vi "student_receiver.vi"() -> ()   [LabVIEW 2021]
uses:
  <vilib>/sound2/lvsound2.llb/Sound Data Format.ctl
  <vilib>/addons/Modulation/Analog/support/mod_Set Error Source.vi
  <vilib>/addons/Modulation/Digital/Support/Common/Validators/mod_Generate Filter Coefficients Validate.vi
  <vilib>/addons/Modulation/Digital/General/subVIs/mod_Generate Filter Coefficients.vi
  <vilib>/addons/Modulation/Digital/General/MT Generate PSK System Parameters(M).vi
  <instrlib>/niUSRP/niUSRP Fetch Rx Data (CDB Cluster).vi
  <vilib>/sound2/lvsound2.llb/Sound File Info (path).vi
  <vilib>/addons/Modulation/niDMT.lvlib
panel:
  in  "stop 2":bool
  out "data":waveform(dbl)[](array[waveform])
  in  "samples per symbol (16)":i32=16
  in  "differential PSK":enum16{"disable", "enable"}(ring)
  out "sound format":T1={"sample rate (S/s)"=22050.0, "number of channels"=2, "bits per sample"=16}
  in  "matched samples per symbol (16)":i32=16
  in  "Path input":path
  out "Constellation Graph":T2(graph)
  in  "pulse shaping samples per symbol (16)":i32=16
  in  "pulse shaping filter (none)":T3(ring)
  out "coerced gain":dbl format="%#_6f"
  out "coerced carrier frequency":dbl=100000.0 format="%#_6p"
  out "coerced IQ rate":dbl=100000.0 format="%#_6p"
  in  "Recv carrier frequency":dbl=100000.0 format="%#_6p"
  in  "Recv IQ rate":dbl=100000.0 format="%#_6p"
  in  "number of samples":i64=100000
  in  "active antenna 2":string
  in  "gain":dbl format="%#_6f"
  out "error out":errorcluster
  in  "error in (no error)":errorcluster
  in  "USRP IP Address":refnum<k15>
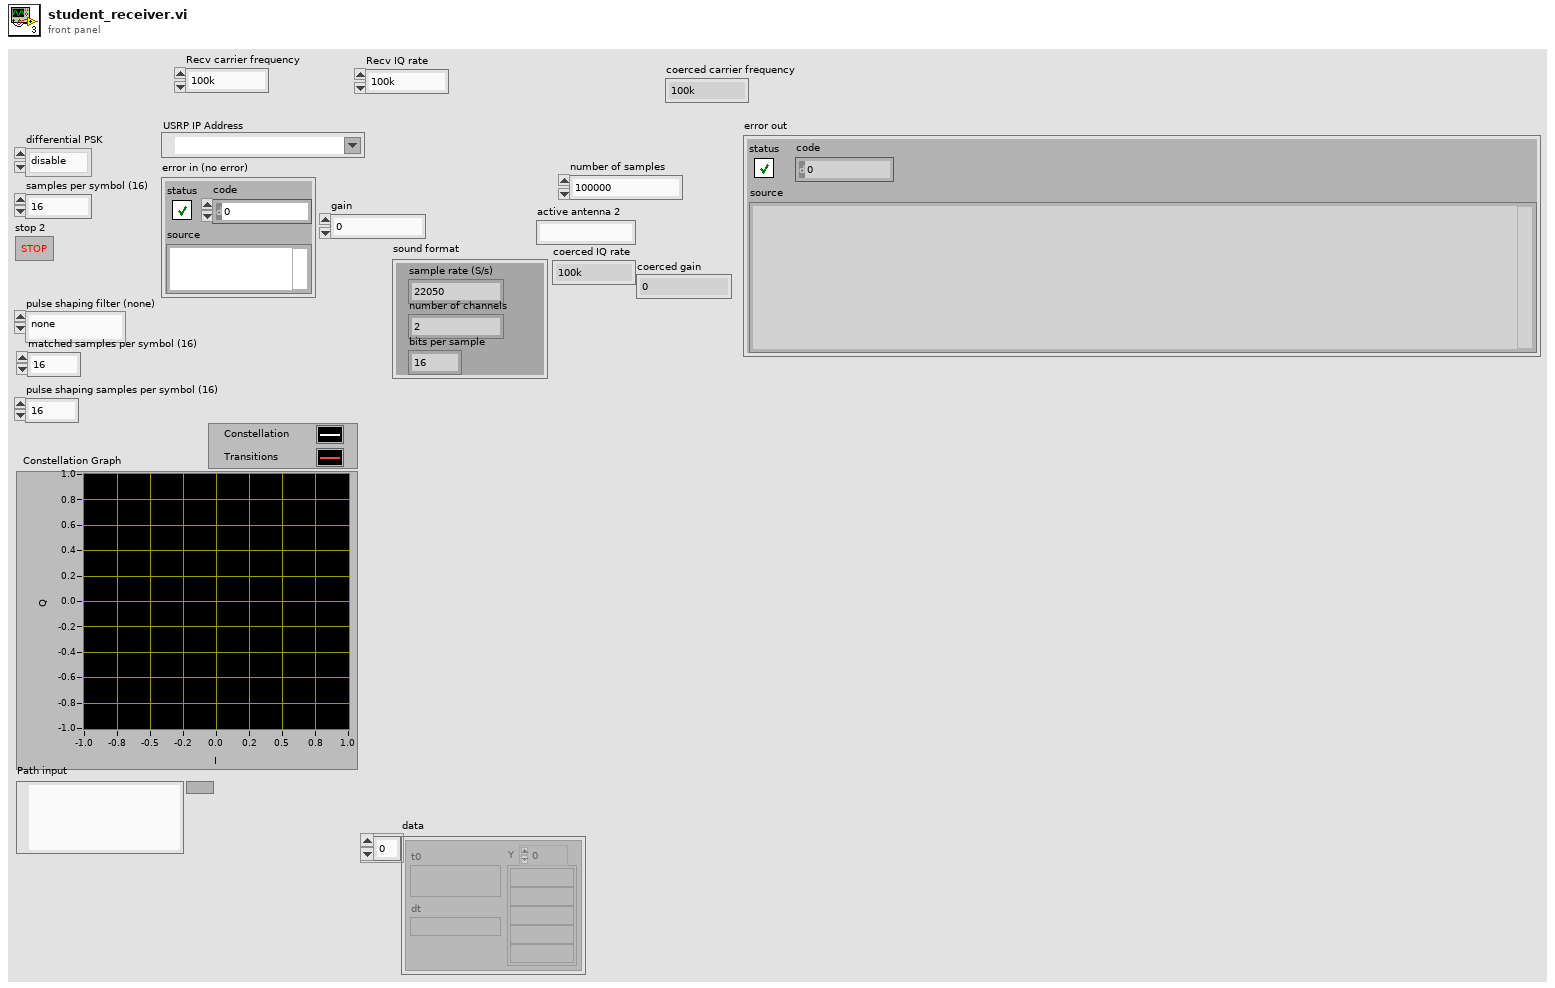
[diagram p1: front panel]
types:
  T1 = typedef "Sound Data Format.ctl" = cluster{"sample rate (S/s)":dbl, "number of channels":i32, "bits per sample":i32}
  T2 = cluster{"Decimated Array":dbl[], "Decimated Array":dbl[]}[]
  T3 = enum16{"none", "Raised Cosine", "Root Raised Cos", "Gaussian"}
  T4 = enum16{"FSK", "PSK", "QAM", "MSK", "PAM", "ASK", "CPM"}
  T5 = cluster{"samples per symbol (16)":i32, "symbol map":cdb[], "differential PSK":enum16{"disable", "enable"}, "PSK type":u16}
  T6 = cluster{"constellation":dbl[], "oversampled data":dbl[]}[]
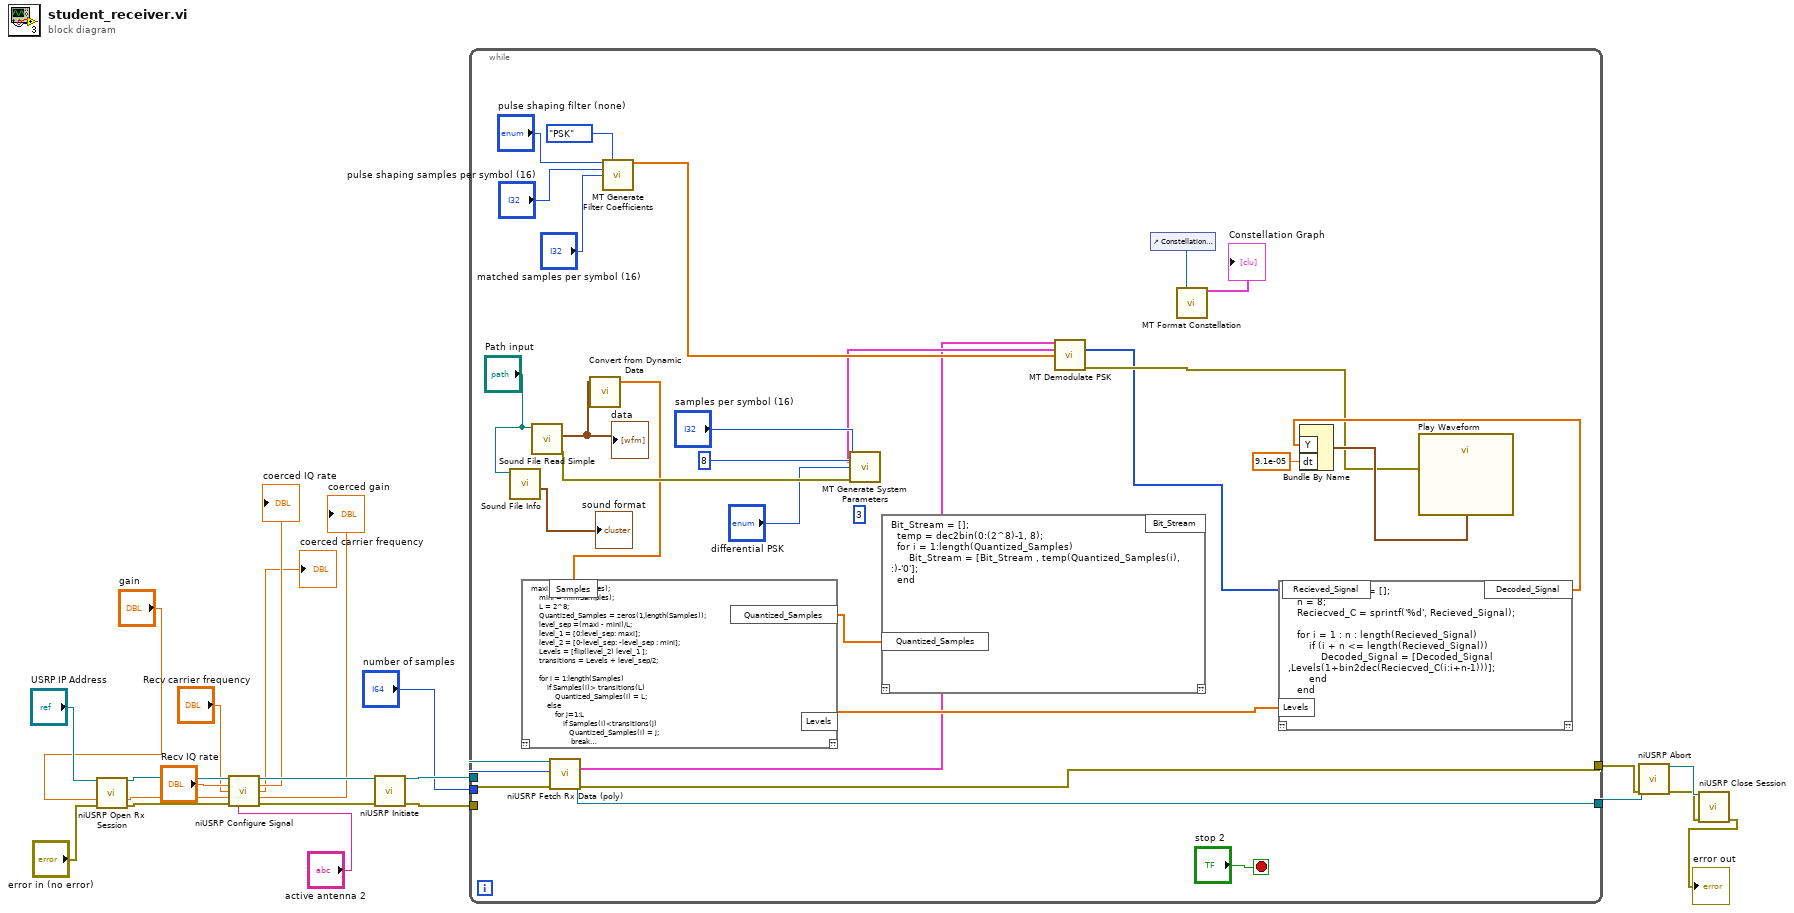
[diagram p0: block diagram]
diagram:
  n1 = call <instrlib>:"niUSRP Open Rx Session.vi"("device names"="USRP IP Address", "error in (no error)"="error in (no error)") -> ("session handle out"=w19:refnum<k15>, "error out"=w18:errorcluster)  [unwired: 12 in]
  n2 = call <instrlib>:"niUSRP Configure Signal.vi"("session handle"=w19, "IQ rate"="Recv IQ rate", "carrier frequency"="Recv carrier frequency", "gain"="gain", "error in (no error)"=w18, "active antenna"="active antenna 2") -> ("session handle out"=w15:refnum<k15>, "coerced IQ rate"=→"coerced IQ rate":dbl, "coerced carrier frequency"=→"coerced carrier frequency":dbl, "coerced gain"=→"coerced gain":dbl, "error out"=w14:errorcluster)  [unwired: 5 in]
  n3 = call <instrlib>:"niUSRP Initiate.vi"("session handle"=w15, "error in (no error)"=w14) -> ("session handle out"=w13:refnum<k15>, "error out"=w12:errorcluster)  [unwired: 12 in]
  n4 = while {
    tunnel: w13 -> [w29]
    tunnel: w12 -> [w28]
    tunnel: "number of samples" -> [w22]
    tunnel: [w25] -> w2
    tunnel: [w24] -> w1
    stop <- "stop 2" stop-if-true
    (unwired) 3 ("bits per symbol")
    n5 = call-poly <vilib>:"Sound File Info.vi"("path"="Path input") -> ("sound format"=→"sound format":T1)  [unwired: 7 in, 3 out]
    n6 = call <vilib>:"Sound File Read Simple.vi"("path"="Path input") -> ("error out"=w42:errorcluster, "data"=w35:waveform(dbl)[])  [unwired: 7 in, 2 out]
    "data" <- w35
    n7 = call-poly <instrlib>:"niUSRP Fetch Rx Data (poly).vi"("session handle"=w29, "number of samples"=w22, "error in (no error)"=w28) -> ("session handle out"=w25:refnum<k15>, "data"=w26:cluster{"t0":dbl, "dt":dbl, "Y":cdb[]}, "error out"=w24:errorcluster)  [unwired: 9 in, 1 out]
    n8 = call "Convert from Dynamic Data"("Dynamic Data Type"=w35) -> ("Array"=w34:dbl[])  [unwired: 3 in]
    n9 = script code="maxi = max(Samples);\n    mini = min(Samples);\n    L = 2^8;\n    Quantized_Samples = zeros(1,length(Samples));\n    level_sep =(maxi - mini)/L; \n    level_1 = [0:level_sep: maxi];\n    level_2 = [0-level_sep: -level_sep : mini];\n    Levels = [flip(level_2) level_1 ];\n    transitions = Levels + level_sep/2;\n    \n    for i = 1:length(Samples)\n        if Samples(i)> transitions(L)\n            Quantized_Samples(i) = L;\n        else\n            for j=1:L\n                if Samples(i)<transitions(j)\n                   Quantized_Samples(i) = j;\n                    break\n                end\n            end\n        end\n    end"("Samples"=w34) -> ("Quantized_Samples"=w36:dbl[], "Levels"=w37:dbl[])  [unwired: 1 in, 1 out]
    n10 = call <vilib>:"MT Generate Filter Coefficients.vi"("pulse shaping filter (none)"="pulse shaping filter (none)", "modulation type"=T4."PSK", "pulse shaping samples per symbol (16)"="pulse shaping samples per symbol (16)", "matched samples per symbol (16)"="matched samples per symbol (16)") -> ("pulse shaping filter coefficients"=w47:dbl[])  [unwired: 9 in, 2 out]
    n11 = call-poly <vilib>:"MT Generate System Parameters.vi"("samples per symbol (16)"="samples per symbol (16)", "M-PSK (4)"=8, "differential PSK"="differential PSK", "error in (no error)"=w42) -> ("PSK system parameters"=w38:T5)  [unwired: 9 in, 2 out]
    n12 = script code="Bit_Stream = [];\n  temp = dec2bin(0:(2^8)-1, 8);  \n  for i = 1:length(Quantized_Samples)\n      Bit_Stream = [Bit_Stream , temp(Quantized_Samples(i), :)-'0'];\n  end"("Quantized_Samples"=w36) -> ()  [unwired: 1 in, 2 out]
    n13 = call <vilib>:"MT Demodulate PSK.vi"("input complex waveform"=w26, "PSK system parameters"=w38, "matched filter coefficients"=w47) -> ("output bit stream"=w27:i8[], "error out"=w30:errorcluster)  [unwired: 8 in, 3 out]
    n14 = control-ref of="Constellation Graph"() -> (w49:refnum<vi>)
    n15 = call <vilib>:"MT Format Constellation.vi"("constellation reference"=w49) -> ("constellation graph"=→"Constellation Graph":T6)  [unwired: 4 in, 10 out]
    n16 = script code="Decoded_Signal = [];\n   n = 8;\n   Reciecved_C = sprintf('%d', Recieved_Signal);\n   \n   for i = 1 : n : length(Recieved_Signal)\n       if (i + n <= length(Recieved_Signal))\n           Decoded_Signal = [Decoded_Signal ,Levels(1+bin2dec(Reciecved_C(i:i+n-1)))];\n       end\n   end"("Recieved_Signal"=w27, "Levels"=w37) -> ("Decoded_Signal"=w33:dbl[])  [unwired: 1 in, 1 out]
    n17 = Bundle By Name("Y"=w33, "dt"=9.1e-05) -> (w32:waveform(dbl))  [unwired: 1 in]
    n18 = call "Play Waveform"("Data"=w32, "error in"=w30) -> ()  [unwired: 17 in, 1 out]
  }
  n19 = call <instrlib>:"niUSRP Abort.vi"("session handle"=w2, "error in (no error)"=w1) -> ("session handle out"=w10:refnum<k15>, "error out"=w9:errorcluster)  [unwired: 12 in]
  n20 = call <instrlib>:"niUSRP Close Session.vi"("session handle"=w10, "error in (no error)"=w9) -> ("error out"=→"error out":errorcluster)  [unwired: 13 in]
